vi "pf_Check_PeakDetect_Mode.vi"(8 "error in":errorcluster, 11 "IMAQ Session in":refnum<k11>) -> (0 "error out":errorcluster, 2 "PeakDetector_Mode":T1, 3 "IMAQ Session out":refnum<k11>)   [LabVIEW 2025, in "Photonfocus_Toolkit.lvlib"]
uses:
  Photonfocus_Toolkit.lvlib
  Controls/pf_PeakDetector_Mode.ctl
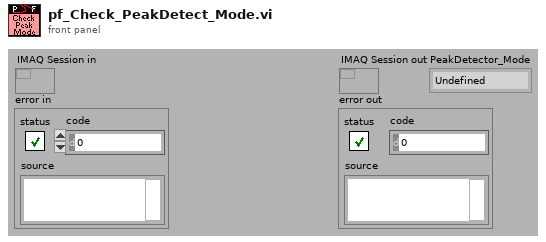
[diagram p1: front panel]
types:
  T1 = typedef "Photonfocus_Toolkit.lvlib/pf_PeakDetector_Mode.ctl" = enum16{"Undefined", "2D only", "2D and 3D", "3D only"}
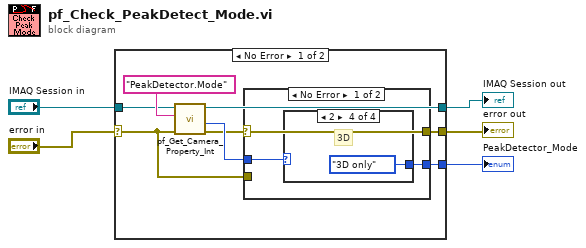
[diagram p0: block diagram]
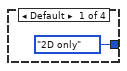
[diagram p2: hidden frame]
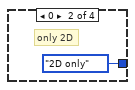
[diagram p3: hidden frame]
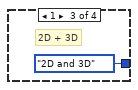
[diagram p4: hidden frame]
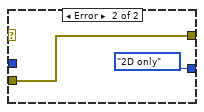
[diagram p5: hidden frame]
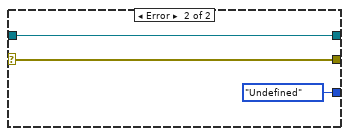
[diagram p6: hidden frame]
diagram:
  n1 = case shown="No Error" "error in" {
    selector: "error in" -> [w6 w25]
    tunnel: "IMAQ Session in" -> [w11 w23]
    tunnel: [w10 w23] -> w4
    tunnel: [w9 pf_PeakDetector_Mode."Undefined" ("PeakDetector_Mode")] -> w1
    tunnel: [w7 w25] -> w2
    frame No Error {
      n2 = call "pf_Get_Camera_Property_Int.vi"("error in (no error)"=w6, "Property Name"="PeakDetector.Mode" ("pProperty"), "IMAQ Session in"=w11) -> ("error out"=w8:errorcluster, "Property Value"=w12:i32, "IMAQ Session out"=w10:refnum<k11>)  [unwired: 6 out]
      n3 = case shown="No Error" w8 {
        selector: w8 -> [w14 _]
        tunnel: w12 -> [w16 _]
        tunnel: [w15 pf_PeakDetector_Mode."2D only" ("PeakDetector_Mode")] -> w9
        tunnel: [w14 w21] -> w7
        tunnel: w6 -> [_ w21]
        frame No Error {
          n4 = case shown="2" w16 {
            tunnel: [pf_PeakDetector_Mode."2D only" ("PeakDetector_Mode") pf_PeakDetector_Mode."2D only" ("PeakDetector_Mode") pf_PeakDetector_Mode."2D and 3D" ("PeakDetector_Mode") pf_PeakDetector_Mode."3D only" ("PeakDetector_Mode")] -> w15
            frame Default {
            }
            frame 0 {
              # "only 2D"
            }
            frame 1 {
              # "2D + 3D"
            }
            frame 2 {
              # "3D"
            }
          }
        }
        frame Error {
        }
      }
    }
    frame Error {
    }
  }
  "IMAQ Session out" <- w4
  "error out" <- w2
  "PeakDetector_Mode" <- w1
